vi "Logging Example.vi"() -> ()   [LabVIEW 2018]
uses:
  api/Log Levels.ctl
  a9dd435e-dc1e-43b6-b577-36eb94796824.vi
  f372ecbb-e024-4756-9563-fbd69adc36fc.vi
  api/configuration/handlers/file_handler/File Handler.lvclass
  C:/Users/Colin/Documents/software_projects/glog/src/api/extension/formatting_handler_interface/Formatting Handler.lvclass
  api/logger_class/Logger.lvclass
  api/Logging.lvlib
panel:
  out "time per iteration (ms)":dbl
  in  "iterations":i32=100
  out "total time (ms)":u32
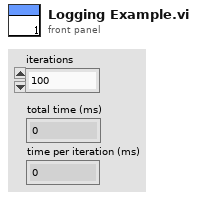
[diagram p1: front panel]
types:
  T1 = typedef "Logging.lvlib/Log Levels.ctl" = enum16{"Trace", "Debug", "Info", "Warning", "Error", "Critical"}
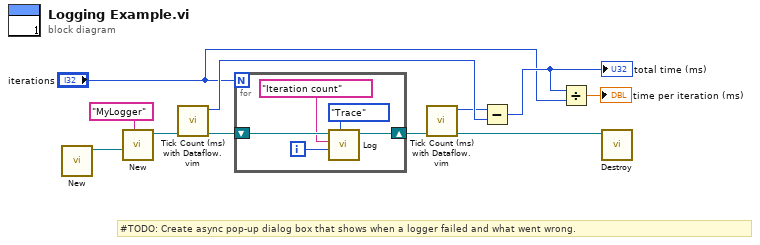
[diagram p0: block diagram]
diagram:
  # "#TODO: Create async pop-up dialog box that shows when a logger failed and what went wrong."
  n1 = call "New.vi"() -> ("file handler"=w11:refnum<class "File Handler.lvclass">)  [unwired: 11 in]
  n2 = call "New.vi"("name (\"Default\")"="MyLogger" ("name"), "log handler (file handler)"=w11) -> ("logger"=w9:refnum<class "Logger.lvclass">)  [unwired: 8 in, 1 out]
  n3 = call "Tick Count (ms) with Dataflow.vim"("dataflow in"=w9) -> ("dataflow out"=w8:refnum<class "Logger.lvclass">, "millisecond timer value"=w6:u32)  [unwired: 9 in]
  n4 = for {
    N: "iterations" -> [_]
    shift-right: [w13] -> w10
    shift-left: w8 -> [w16]
    i -> [w12]
    n5 = call "Log.vi"("log level"=Log_Levels."Trace" ("level"), "data (null)"=w12, "message"="Iteration count", "logger in"=w16) -> ("logger out"=w13:refnum<class "Logger.lvclass">)  [unwired: 7 in]
  }
  n6 = call "Tick Count (ms) with Dataflow.vim"("dataflow in"=w10) -> ("dataflow out"=w7:refnum<class "Logger.lvclass">, "millisecond timer value"=w5:u32)  [unwired: 9 in]
  n7 = Subtract(x=w5, y=w6) -> (x-y=w4:u32)
  "total time (ms)" <- w4
  n8 = Divide(x=w4, y="iterations") -> (x/y=→"time per iteration (ms)":dbl)
  n9 = call "Destroy.vi"("logger in"=w7) -> ()  [unwired: 9 in, 2 out]
